vi "AddObserver.vi"(8 "error in (no error)":errorcluster, 10 "ObserverNotifierReference":refnum<notifier>, 11 "Observable in":refnum<class "Observable.lvclass">) -> (0 "error out":errorcluster, 3 "Observable out":refnum<class "Observable.lvclass">)   [LabVIEW 2013, in "Observable.lvclass"]
uses:
  Observable.lvclass
  Observable.lvclass/Observable.ctl
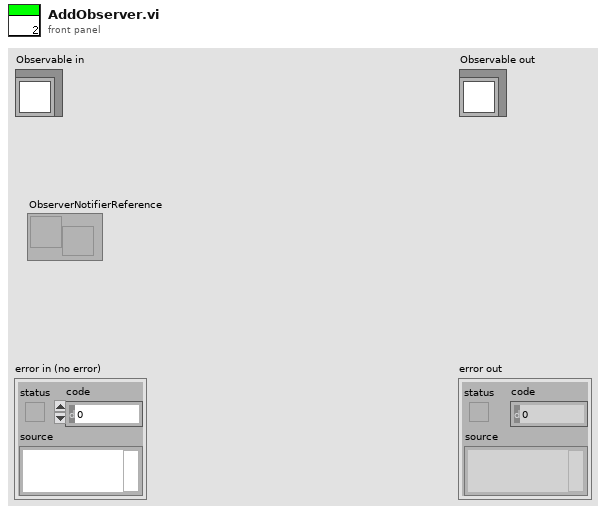
[diagram p1: front panel]
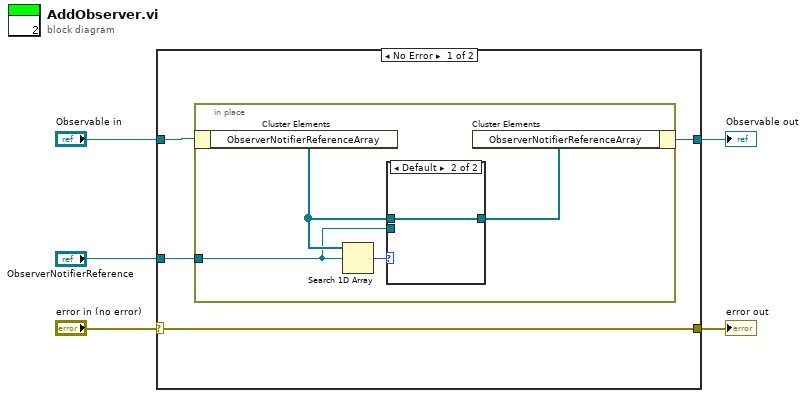
[diagram p0: block diagram]
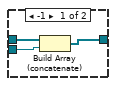
[diagram p2: hidden frame]
diagram:
  n1 = case shown="No Error" "error in (no error)" {
    selector: "error in (no error)" -> [w6 w19]
    tunnel: [w6 w19] -> w4
    tunnel: [w7 w18] -> w2
    tunnel: "Observable in" -> [w8 w18]
    tunnel: "ObserverNotifierReference" -> [w9 _]
    frame No Error {
      n2 = in-place {
        in-place-border: w9 -> [w10]
        n3 = in-place-cluster #1(w8) -> ("ObserverNotifierReferenceArray"=w11:refnum<notifier>[])
        n4 = Search 1D Array(1D array=w11, element=w10) -> (index of element=w12:i32)  [unwired: 1 in]
        n5 = case shown="Default" w12 {
          tunnel: w11 -> [w16 w17]
          tunnel: [w14 w17] -> w13
          tunnel: w10 -> [w15 _]
          frame -1 {
            n6 = Build Array (concatenate)(w16, w15) -> (w14:refnum<notifier>[])
          }
          frame Default {
          }
        }
        n7 = in-place-cluster #1("ObserverNotifierReferenceArray"=w13) -> (w7:refnum<class "Observable.lvclass">)
      }
    }
    frame Error {
    }
  }
  "error out" <- w4
  "Observable out" <- w2
